vi "MotionProfileTest.vi"() -> ()   [LabVIEW 2017]
panel:
  out "NumPoints":i32
  out "Update Rate (Hz)":dbl
  in  "stop":bool
  out "Motion Profile":T1(graph)
  in  "Starting Position (rotations)":dbl
  in  "Acceleration Ramp Time (ms)":dbl=200.0
  in  "Trajectory Point Interval (ms)":dbl=10.0
  in  "Velocity Ramp Time (ms)":dbl=400.0
  in  "Maximum Travel Speed":dbl=240.0
  in  "Travel Distance (rotations)":dbl=5.0
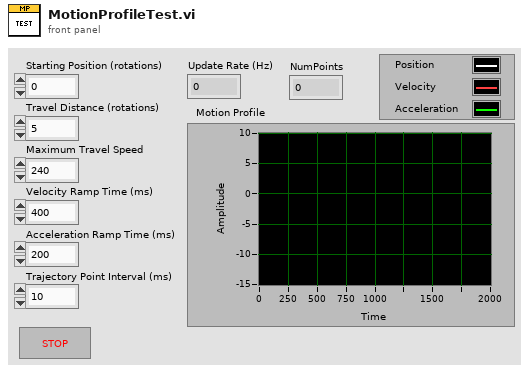
[diagram p1: front panel]
types:
  T1 = cluster{dbl, "Trajectory Point Interval (ms)":dbl, dbl[][]}
  T2 = typedef "TrajectoryPoint.ctl" = cluster{"Position ":dbl, "Velocity ":dbl, "Time (ms)":dbl, "Last Point":bool}
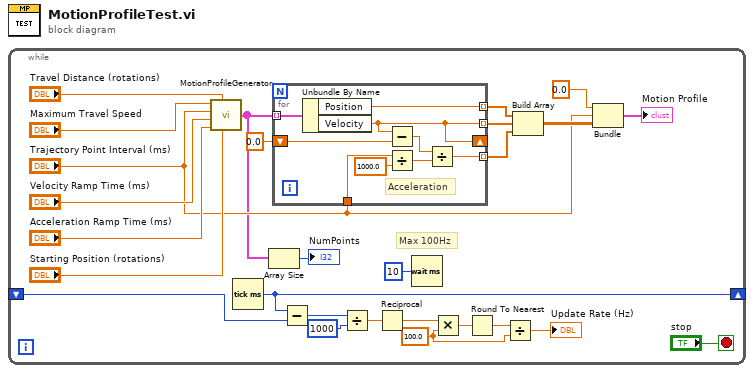
[diagram p0: block diagram]
diagram:
  n1 = while {
    shift-right: [w12] -> _
    shift-left: _ -> [w13]
    stop <- "stop" stop-if-true
    w5 = 100.0 ("y")
    # "Max 100Hz"
    n2 = call "MotionProfileGenerator.vi"("Starting Position (rotations)"="Starting Position (rotations)", "Travel Distance (rotations)"="Travel Distance (rotations)", "Acceleration Ramp Time (ms)"="Acceleration Ramp Time (ms)", "Velocity Ramp Time (ms)"="Velocity Ramp Time (ms)", "Trajectory Point Interval (ms)"="Trajectory Point Interval (ms)", "Maximum Travel Speed (rpm)"="Maximum Travel Speed") -> ("Trajectory Points"=w2:T2[])
    n3 = Tick Count (ms)() -> (millisecond timer value=w12:u32)
    n4 = Array Size(array=w2) -> (size(s)=→"NumPoints":i32)
    n5 = for {
      tunnel: w2 -> [w36] mode=indexing
      tunnel: [w35] -> w20 mode=indexing
      tunnel: [w34] -> w19 mode=indexing
      shift-right: [w34] -> _
      shift-left: 0.0 ("Velocity") -> [w33]
      tunnel: [w31] -> w16 mode=indexing
      tunnel: "Trajectory Point Interval (ms)" -> [w30]
      # "Acceleration"
      n6 = Unbundle By Name(w36) -> ("Position"=w35:dbl, "Velocity"=w34:dbl)
      n7 = Subtract(x=w34, y=w33) -> (x-y=w32:dbl)
      n8 = Divide(x=w30, y=1000.0) -> (x/y=w28:dbl)
      n9 = Divide(x=w32, y=w28) -> (x/y=w31:dbl)
    }
    n10 = Subtract(x=w12, y=w13) -> (x-y=w11:u32)
    n11 = Divide(x=w11, y=u32 1000) -> (x/y=w9:dbl)
    n12 = Reciprocal(x=w9) -> (1/x=w8:dbl)
    n13 = Wait (ms)(milliseconds to wait=u32 10) -> ()  [unwired: 1 out]
    n14 = Multiply(x=w8, y=w5) -> (x*y=w7:dbl)
    n15 = Round To Nearest(number=w7) -> (nearest integer value=w6:dbl)
    n16 = Divide(x=w6, y=w5) -> (x/y=→"Update Rate (Hz)":dbl)
    n17 = Build Array(w20, w19, w16) -> (w18:dbl[][])
    n18 = Bundle(0.0, "Trajectory Point Interval (ms)"="Trajectory Point Interval (ms)", w18) -> (→"Motion Profile":T1)  [unwired: 1 in]
  }
